vi "Enqueue Message (Array).vi"(6 "Priority Message? Array":bool[](array[boolean]), 8 "error in (no error)":errorcluster, 10 "Message Array":string[](array[string]), 11 "Message Queue":refnum<queue>) -> (0 "error out":errorcluster, 3 "dup Message Queue":refnum<queue>)   [LabVIEW 2025, in "LAB-IQ Message Queue.lvlib"]
doc: "For a regular message, enqueue the message. For a priority message, enqueue it at the front of the queue."
uses:
  LAB-IQ Message Queue.lvlib
  Message Cluster.ctl
panel:
  in  "output data":dbl[][](array[numeric])
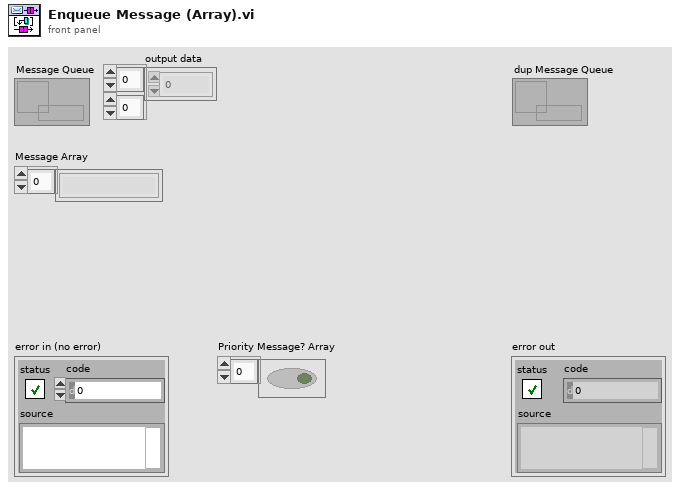
[diagram p1: front panel]
types:
  T1 = typedef "LAB-IQ Message Queue.lvlib/Message Cluster.ctl" = cluster{"Message":string, "output data":dbl[][]}
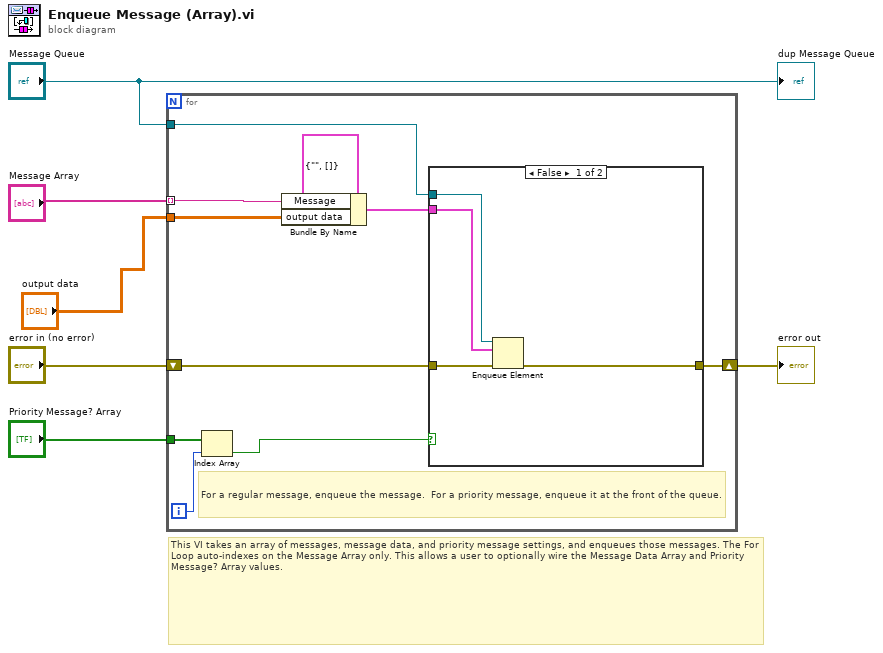
[diagram p0: block diagram]
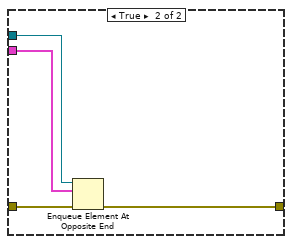
[diagram p2: hidden frame]
diagram:
  # "This VI takes an array of messages, message data, and priority message settings, and enqueues those messages. The For Loop auto-indexes on the Message Array only. This allows a user to optionally wire the Message Data Array and Priority Message? Array values."
  n1 = for {
    tunnel: "Message Array" -> [w15] mode=indexing
    tunnel: "output data" -> [w7]
    tunnel: "Priority Message? Array" -> [w10]
    tunnel: "Message Queue" -> [w12]
    shift-right: [w13] -> w3
    shift-left: "error in (no error)" -> [w14]
    i -> [w8]
    # "For a regular message, enqueue the message.  For a priority message, enqueue it at the front of the queue."
    n2 = Index Array(array=w10, index=w8) -> (element=w9:bool)
    n3 = Bundle By Name(cluster=T1 {"Message"="", "output data"=[]} ("Message Cluster"), "Message"=w15, "output data"=w7) -> (w11:T1)
    n4 = case shown="False" w9 {
      tunnel: w14 -> [w20 w24]
      tunnel: [w19 w23] -> w13
      tunnel: w12 -> [w18 w22]
      tunnel: w11 -> [w17 w21]
      frame False {
        n5 = Enqueue Element(queue=w18, element=w17, error in (no error)=w20) -> (error out=w19:errorcluster)  [unwired: 1 in, 2 out]
      }
      frame True {
        n6 = Enqueue Element At Opposite End(queue=w22, element=w21, error in (no error)=w24) -> (error out=w23:errorcluster)  [unwired: 1 in, 2 out]
      }
    }
  }
  "error out" <- w3
  "dup Message Queue" <- "Message Queue"
